vi "findVales.vi"(7 "#_foundPeaks":i32, 8 "Error In":errorcluster, 9 "VE_E":dbl[](array[numeric]), 10 "iPeaksLocation":dbl[](array[numeric]), 11 "filteredSignal":dbl[](array[numeric])) -> (0 "Error Out":errorcluster, 2 "valesAmplitude":dbl[](array[numeric]), 3 "iValesLocation":dbl[](array[numeric]))   [LabVIEW 2012]
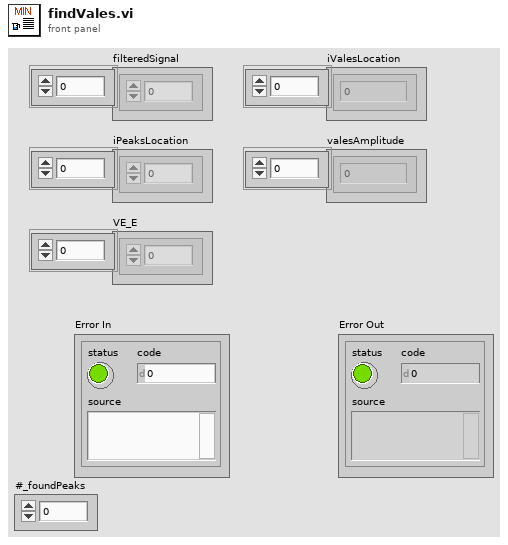
[diagram p1: front panel]
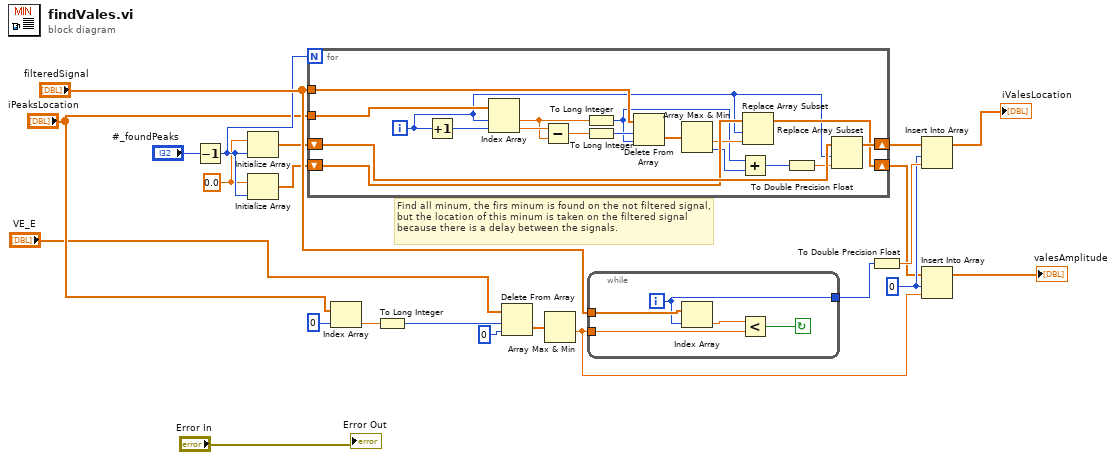
[diagram p0: block diagram]
diagram:
  w15 = 0 ("index")
  w9 = 0.0 ("element")
  # "Find all minum, the firs minum is found on the not filtered signal, but the location of this minum is taken on the filtered signal because there is a delay between the signals."
  n1 = Decrement(x="#_foundPeaks") -> (x-1=w16:i32)
  n2 = Initialize Array(w9, w16) -> (w11:dbl[])
  n3 = Initialize Array(w9, w16) -> (w10:dbl[])
  n4 = for {
    N: w16 -> [_]
    tunnel: "filteredSignal" -> [w40]
    tunnel: "iPeaksLocation" -> [w39]
    shift-right: [w31] -> w14
    shift-left: w11 -> [w32]
    shift-right: [w29] -> w13
    shift-left: w10 -> [w30]
    i -> [w28]
    n5 = Increment(x=w28) -> (x+1=w38:i32)
    n6 = Index Array(array=w39, index #1=w28, index #2=w38) -> (element #1=w36:dbl, element #2=w37:dbl)
    n7 = Subtract(x=w37, y=w36) -> (x-y=w35:dbl)
    n8 = To Long Integer(number=w36) -> (32bit integer=w23:i32)
    n9 = To Long Integer(number=w35) -> (32bit integer=w34:i32)
    n10 = Delete From Array(array=w40, length=w34, index=w23) -> (deleted portion=w33:dbl[])  [unwired: 1 out]
    n11 = Array Max & Min(array=w33) -> (min value=w27:dbl, min index (indices)=w26:i32)  [unwired: 2 out]
    n12 = Add(x=w23, y=w26) -> (x+y=w24:i32)
    n13 = Replace Array Subset(array=w30, new element=w27, index=w28) -> (w29:dbl[])
    n14 = To Double Precision Float(number=w24) -> (double precision float=w25:dbl)
    n15 = Replace Array Subset(array=w32, new element=w25, index=w28) -> (w31:dbl[])
  }
  n16 = Index Array(array="iPeaksLocation", index=0) -> (element=w5:dbl)
  n17 = To Long Integer(number=w5) -> (32bit integer=w20:i32)
  n18 = Delete From Array(array="VE_E", length=w20, index=0) -> (deleted portion=w7:dbl[])  [unwired: 1 out]
  n19 = Array Max & Min(array=w7) -> (min value=w18:dbl)  [unwired: 3 out]
  n20 = while {
    tunnel: w18 -> [w43]
    tunnel: "filteredSignal" -> [w45]
    tunnel: [w41] -> w21
    i -> [w41]
    stop <- w42 continue-if-true
    n21 = Index Array(array=w45, index=w41) -> (element=w44:dbl)
    n22 = Less?(x=w44, y=w43) -> (x < y?=w42:bool)
  }
  n23 = To Double Precision Float(number=w21) -> (double precision float=w22:dbl)
  n24 = Insert Into Array(array=w14, index=w15, new element=w22) -> (→"iValesLocation":dbl[])
  n25 = Insert Into Array(array=w13, index=w15, new element=w18) -> (→"valesAmplitude":dbl[])
  "Error Out" <- "Error In"
